vi "solar_type Set Value (ASCII).vi"(6 "ArrayDelimiters (1D,2D)":string[](array[string]), 7 "Keep Attributes? (F)":bool, 8 "error in (no error)":errorcluster, 10 "Value (ASCII)":string, 11 "Variant":variant) -> (0 "error out":errorcluster, 2 "Value (Binary)":string, 3 "Variant out":variant)   [LabVIEW 2018]
doc: "This sets the ASCII value into the Variant data."
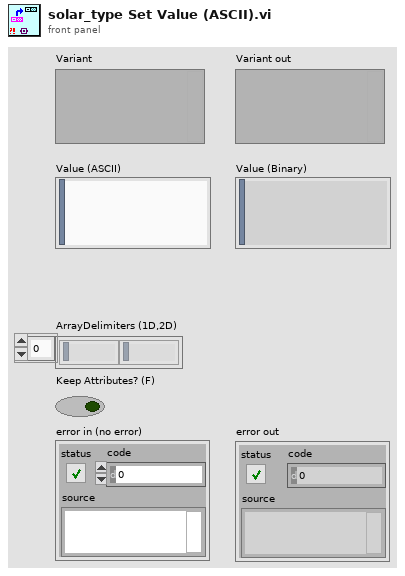
[diagram p1: front panel]
types:
  T1 = typedef "solar_type Item Type.ctl" = enum16{"NULL", "UNKNOWN", "CLUSTER", "I8", "I16", "I32", "I64", "U8", "U16", "U32", "U64", "U8_ENUM", "U16_ENUM", "U32_ENUM", "SGL", "DBL", "BOOLEAN", "STRING", "PATH", "VISA", "TAG", "TIME", "I8_1D", "I16_1D", "I32_1D", "I64_1D", "U8_1D", "U16_1D", "U32_1D", "U64_1D", "U8_ENUM_1D", "U16_ENUM_1D", "U32_ENUM_1D", "SGL_1D", "DBL_1D", "BOOLEAN_1D", "STRING_1D", "PATH_1D", "VISA_1D", "TAG_1D", "TIME_1D", "I8_2D", "I16_2D", "I32_2D", "I64_2D", "U8_2D", "U16_2D", "U32_2D", "U64_2D", "U8_ENUM_2D", "U16_ENUM_2D", "U32_ENUM_2D", "SGL_2D", "DBL_2D", "BOOLEAN_2D", "STRING_2D", "PATH_2D", "VISA_2D", "TAG_2D", "TIME_2D"}
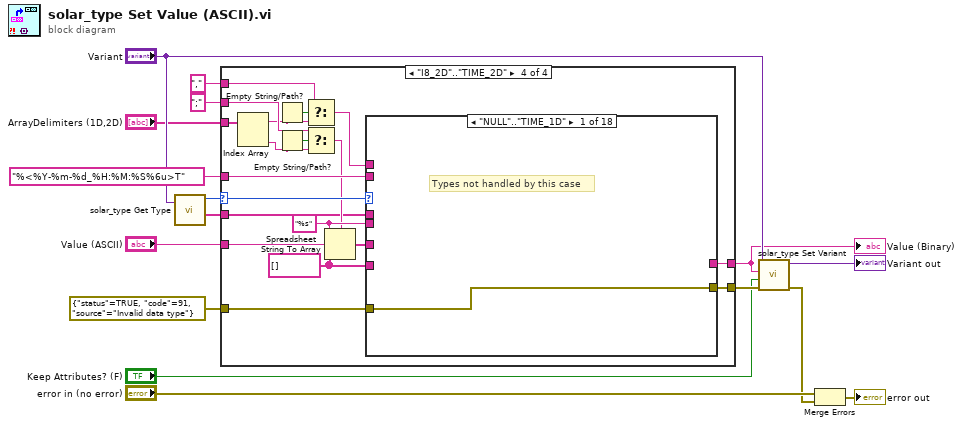
[diagram p0: block diagram]
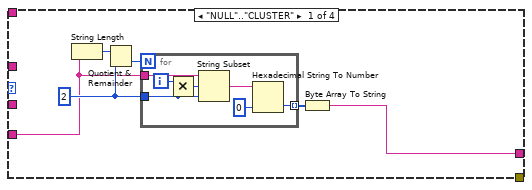
[diagram p2: hidden frame]
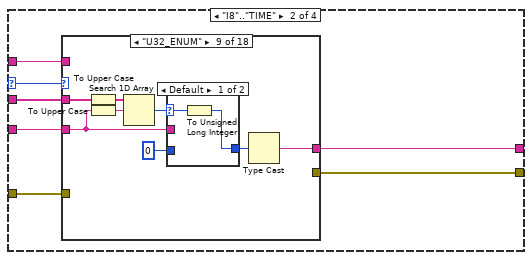
[diagram p3: hidden frame]
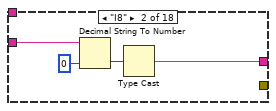
[diagram p5: hidden frame]
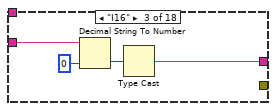
[diagram p6: hidden frame]
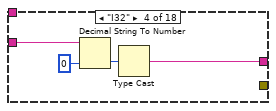
[diagram p7: hidden frame]
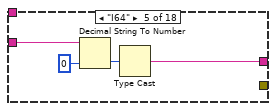
[diagram p8: hidden frame]
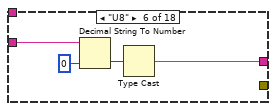
[diagram p9: hidden frame]
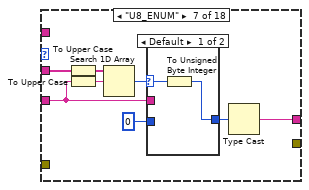
[diagram p10: hidden frame]
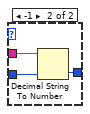
[diagram p11: hidden frame]
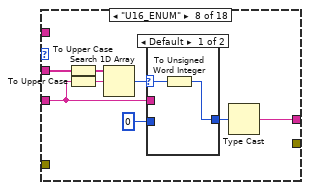
[diagram p12: hidden frame]
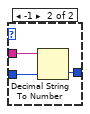
[diagram p13: hidden frame]
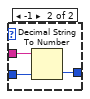
[diagram p14: hidden frame]
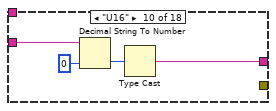
[diagram p15: hidden frame]
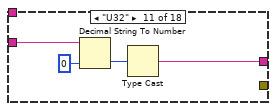
[diagram p16: hidden frame]
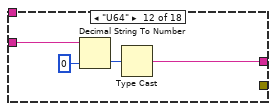
[diagram p17: hidden frame]
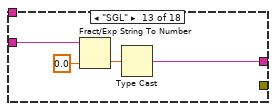
[diagram p18: hidden frame]
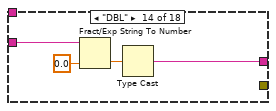
[diagram p19: hidden frame]
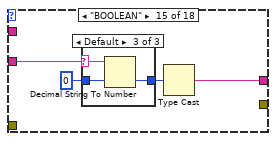
[diagram p20: hidden frame]
diagram:
  n1 = call "solar_type Get Type.vi"("Variant"="Variant") -> ("Type"=w11:T1, "Enum Names"=w3:string[])  [unwired: 4 in, 1 out]
  n2 = case shown="\"I8_2D\"..\"TIME_2D\"" w11 {
    selector: w11 -> [_ w36 w154 w300]
    tunnel: "Value (ASCII)" -> [w18 w31 w150 w299]
    tunnel: [_ w33 w151 w302] -> w10
    tunnel: [w17 w35 w153 w303] -> w1
    tunnel: errorcluster {"status"=TRUE, "code"=91, "source"="Invalid data type"} ("error in (no error)") -> [_ w34 w152 w301]
    tunnel: "%<%Y-%m-%d_%H:%M:%S%6u>T" -> [_ w32 w146 w298]
    tunnel: "," -> [_ _ w143 w295]
    tunnel: ";" -> [_ _ _ w292]
    tunnel: w3 -> [_ w30 w140 w288]
    tunnel: "ArrayDelimiters (1D,2D)" -> [_ _ w141 w290]
    frame "NULL".."CLUSTER" {
      w22 = 2 ("y")
      n3 = String Length(string=w18) -> (length=w20:i32)
      n4 = Quotient & Remainder(x=w20, y=w22) -> (floor(x/y)=w21:i32)  [unwired: 1 out]
      n5 = for {
        N: w21 -> [_]
        tunnel: w18 -> [w29]
        tunnel: [w24] -> w19 mode=indexing
        tunnel: w22 -> [w23]
        i -> [w28]
        n6 = Multiply(x=w28, y=w23) -> (x*y=w27:i32)
        n7 = String Subset(string=w29, offset (0)=w27, length (rest)=w23) -> (substring=w26:string)
        n8 = Hexadecimal String To Number(string=w26, default (0uL)=u8 0 ("default (0 U32)")) -> (number=w24:u8)  [unwired: 1 in, 1 out]
      }
      n9 = Byte Array To String(unsigned byte array=w19) -> (string=w17:string)
    }
    frame "I8".."TIME" {
      n10 = case shown="\"U32_ENUM\"" w36 {
        tunnel: w31 -> [_ w41 w45 w49 w53 w57 w62 w75 w88 w100 w104 w108 w112 w116 w120 w127 w131 w139]
        tunnel: [_ w38 w42 w46 w50 w54 w64 w77 w90 w97 w101 w105 w109 w113 w117 w126 w133 w134] -> w35
        tunnel: w34 -> [w37 _ _ _ _ _ _ _ _ _ _ _ _ _ _ _ _ _]
        tunnel: [w37 _ _ _ _ _ _ _ _ _ _ _ _ _ _ _ w132 w138] -> w33
        tunnel: w32 -> [_ _ _ _ _ _ _ _ _ _ _ _ _ _ _ _ _ w137]
        tunnel: w30 -> [_ _ _ _ _ _ w63 w76 w89 _ _ _ _ _ _ _ _ _]
        frame "NULL".."CLUSTER", "I8_1D".."TIME_2D" {
          # "Not handled by this case"
        }
        frame "I8" {
          n11 = Decimal String To Number(string=w41, default (0L)=i8 0 ("default (0 I32)")) -> (number=w39:i8)  [unwired: 1 in, 1 out]
          n12 = Type Cast(x=w39) -> (*(type *) &x=w38:string)  [unwired: 1 in]
        }
        frame "I16" {
          n13 = Decimal String To Number(string=w45, default (0L)=i16 0 ("default (0 I32)")) -> (number=w43:i16)  [unwired: 1 in, 1 out]
          n14 = Type Cast(x=w43) -> (*(type *) &x=w42:string)  [unwired: 1 in]
        }
        frame "I32" {
          n15 = Decimal String To Number(string=w49, default (0L)=0 ("default (0 I32)")) -> (number=w47:i32)  [unwired: 1 in, 1 out]
          n16 = Type Cast(x=w47) -> (*(type *) &x=w46:string)  [unwired: 1 in]
        }
        frame "I64" {
          n17 = Decimal String To Number(string=w53, default (0L)=i64 0 ("default (0 I32)")) -> (number=w51:i64)  [unwired: 1 in, 1 out]
          n18 = Type Cast(x=w51) -> (*(type *) &x=w50:string)  [unwired: 1 in]
        }
        frame "U8" {
          n19 = Decimal String To Number(string=w57, default (0L)=u8 0 ("default (0 I32)")) -> (number=w55:u8)  [unwired: 1 in, 1 out]
          n20 = Type Cast(x=w55) -> (*(type *) &x=w54:string)  [unwired: 1 in]
        }
        frame "U8_ENUM" {
          n21 = To Upper Case(1:w63) -> (0:w60:string[])
          n22 = To Upper Case(1:w62) -> (0:w59:string)
          n23 = Search 1D Array(1D array=w60, element=w59) -> (index of element=w61:i32)  [unwired: 1 in]
          n24 = case shown="Default" w61 {
            selector: w61 -> [w67 _]
            tunnel: [w66 w70] -> w65
            tunnel: w62 -> [_ w69]
            tunnel: u8 0 ("default (0 I32)") -> [_ w68]
            frame Default {
              n25 = To Unsigned Byte Integer(number=w67) -> (unsigned 8bit integer=w66:u8)
            }
            frame -1 {
              n26 = Decimal String To Number(string=w69, default (0L)=w68) -> (number=w70:u8)  [unwired: 1 in, 1 out]
            }
          }
          n27 = Type Cast(x=w65) -> (*(type *) &x=w64:string)  [unwired: 1 in]
        }
        frame "U16_ENUM" {
          n28 = To Upper Case(1:w76) -> (0:w73:string[])
          n29 = To Upper Case(1:w75) -> (0:w72:string)
          n30 = Search 1D Array(1D array=w73, element=w72) -> (index of element=w74:i32)  [unwired: 1 in]
          n31 = case shown="Default" w74 {
            selector: w74 -> [w80 _]
            tunnel: [w79 w83] -> w78
            tunnel: w75 -> [_ w82]
            tunnel: u16 0 ("default (0 I32)") -> [_ w81]
            frame Default {
              n32 = To Unsigned Word Integer(number=w80) -> (unsigned 16bit integer=w79:u16)
            }
            frame -1 {
              n33 = Decimal String To Number(string=w82, default (0L)=w81) -> (number=w83:u16)  [unwired: 1 in, 1 out]
            }
          }
          n34 = Type Cast(x=w78) -> (*(type *) &x=w77:string)  [unwired: 1 in]
        }
        frame "U32_ENUM" {
          n35 = To Upper Case(1:w89) -> (0:w86:string[])
          n36 = To Upper Case(1:w88) -> (0:w85:string)
          n37 = Search 1D Array(1D array=w86, element=w85) -> (index of element=w87:i32)  [unwired: 1 in]
          n38 = case shown="Default" w87 {
            selector: w87 -> [w93 _]
            tunnel: [w92 w96] -> w91
            tunnel: w88 -> [_ w95]
            tunnel: u32 0 ("default (0 I32)") -> [_ w94]
            frame Default {
              n39 = To Unsigned Long Integer(number=w93) -> (unsigned 32bit integer=w92:u32)
            }
            frame -1 {
              n40 = Decimal String To Number(string=w95, default (0L)=w94) -> (number=w96:u32)  [unwired: 1 in, 1 out]
            }
          }
          n41 = Type Cast(x=w91) -> (*(type *) &x=w90:string)  [unwired: 1 in]
        }
        frame "U16" {
          n42 = Decimal String To Number(string=w100, default (0L)=u16 0 ("default (0 I32)")) -> (number=w98:u16)  [unwired: 1 in, 1 out]
          n43 = Type Cast(x=w98) -> (*(type *) &x=w97:string)  [unwired: 1 in]
        }
        frame "U32" {
          n44 = Decimal String To Number(string=w104, default (0L)=u32 0 ("default (0 I32)")) -> (number=w102:u32)  [unwired: 1 in, 1 out]
          n45 = Type Cast(x=w102) -> (*(type *) &x=w101:string)  [unwired: 1 in]
        }
        frame "U64" {
          n46 = Decimal String To Number(string=w108, default (0L)=u64 0 ("default (0 I32)")) -> (number=w106:u64)  [unwired: 1 in, 1 out]
          n47 = Type Cast(x=w106) -> (*(type *) &x=w105:string)  [unwired: 1 in]
        }
        frame "SGL" {
          n48 = Fract/Exp String To Number(string=w112, default (0 dbl)=sgl 0.0 ("default (0 I32)")) -> (number=w110:sgl)  [unwired: 2 in, 1 out]
          n49 = Type Cast(x=w110) -> (*(type *) &x=w109:string)  [unwired: 1 in]
        }
        frame "DBL" {
          n50 = Fract/Exp String To Number(string=w116, default (0 dbl)=0.0 ("default (0 I32)")) -> (number=w114:dbl)  [unwired: 2 in, 1 out]
          n51 = Type Cast(x=w114) -> (*(type *) &x=w113:string)  [unwired: 1 in]
        }
        frame "BOOLEAN" {
          n52 = case shown="Default" w120 {
            selector: w120 -> [_ _ w125]
            tunnel: u8 0 ("default (0 I32)") -> [w121 _ w124]
            tunnel: [w121 u8 1 w123] -> w118
            frame "false" {
            }
            frame "true" {
            }
            frame Default {
              n53 = Decimal String To Number(string=w125, default (0L)=w124) -> (number=w123:u8)  [unwired: 1 in, 1 out]
            }
          }
          n54 = Type Cast(x=w118) -> (*(type *) &x=w117:string)  [unwired: 1 in]
        }
        frame "STRING", "VISA", "TAG" {
          n55 = String Length(string=w127) -> (length=w129:i32)
          n56 = Type Cast(x=w129) -> (*(type *) &x=w128:string)  [unwired: 1 in]
          n57 = Concatenate Strings(w128, w127) -> (w126:string)
        }
        frame "PATH" {
          # "PTH0<I32_size>..."
          n58 = String To Path(string=w131) -> (path=w130:path)
          n59 = Flatten To String(anything=w130) -> (data string=w133:string, error out=w132:errorcluster)  [unwired: 3 in, 1 out]
        }
        frame "TIME" {
          # "16 bytes"
          n60 = Scan From String(format string=w137, input string=w139, default 1=timestamp(0 s since 1904-01-01)) -> (error out=w138:errorcluster, output 1=w135:timestamp)  [unwired: 2 in, 2 out]
          n61 = Flatten To String(anything=w135) -> (data string=w134:string)  [unwired: 3 in, 2 out]
        }
      }
    }
    frame "I8_1D".."TIME_1D" {
      n62 = Index Array(array=w141) -> (element=w142:string)  [unwired: 1 in]
      n63 = Empty String/Path?(string/path=w142) -> (empty?=w145:bool)
      n64 = Select(t=w143, s=w145, f=w142) -> (s? t:f=w144:string)
      n65 = Spreadsheet String To Array(delimiter (Tab)=w144, format string="%s", spreadsheet string=w150, array type (2D Dbl)=string[] []) -> (array=w147:string[])
      n66 = case shown="\"U32_ENUM_1D\"" w154 {
        tunnel: w147 -> [_ w158 w163 w168 w173 w178 w183 w188 w193 w197 w214 w231 w249 w254 w260 w269 w273 w280]
        tunnel: [_ w160 w165 w170 w175 w180 w185 w190 w195 w201 w218 w235 w251 w256 w258 w271 w275 w281] -> w153
        tunnel: w152 -> [w155 _ _ _ _ _ _ _ _ _ _ _ _ _ _ _ _ _]
        tunnel: [w155 w159 w164 w169 w174 w179 w184 w189 w194 w200 w217 w234 w250 w255 w257 w270 w274 w279] -> w151
        tunnel: w146 -> [_ _ _ _ _ _ _ _ _ _ _ _ _ _ _ _ _ w278]
        tunnel: w140 -> [_ _ _ _ _ _ _ _ _ w198 w215 w232 _ _ _ _ _ _]
        frame "NULL".."TIME", "I8_2D".."TIME_2D" {
        }
        frame "I8_1D" {
          n67 = Decimal String To Number(string=w158, default (0L)=i8 0 ("default (0 I32)")) -> (number=w156:i8[])  [unwired: 1 in, 1 out]
          n68 = Flatten To String(anything=w156) -> (data string=w160:string, error out=w159:errorcluster)  [unwired: 3 in, 1 out]
        }
        frame "I16_1D" {
          n69 = Decimal String To Number(string=w163, default (0L)=i16 0 ("default (0 I32)")) -> (number=w161:i16[])  [unwired: 1 in, 1 out]
          n70 = Flatten To String(anything=w161) -> (data string=w165:string, error out=w164:errorcluster)  [unwired: 3 in, 1 out]
        }
        frame "I32_1D" {
          n71 = Decimal String To Number(string=w168, default (0L)=0 ("default (0 I32)")) -> (number=w166:i32[])  [unwired: 1 in, 1 out]
          n72 = Flatten To String(anything=w166) -> (data string=w170:string, error out=w169:errorcluster)  [unwired: 3 in, 1 out]
        }
        frame "I64_1D" {
          n73 = Decimal String To Number(string=w173, default (0L)=i64 0 ("default (0 I32)")) -> (number=w171:i64[])  [unwired: 1 in, 1 out]
          n74 = Flatten To String(anything=w171) -> (data string=w175:string, error out=w174:errorcluster)  [unwired: 3 in, 1 out]
        }
        frame "U8_1D" {
          n75 = Decimal String To Number(string=w178, default (0L)=u8 0 ("default (0 I32)")) -> (number=w176:u8[])  [unwired: 1 in, 1 out]
          n76 = Flatten To String(anything=w176) -> (data string=w180:string, error out=w179:errorcluster)  [unwired: 3 in, 1 out]
        }
        frame "U16_1D" {
          n77 = Decimal String To Number(string=w183, default (0L)=u16 0 ("default (0 I32)")) -> (number=w181:u16[])  [unwired: 1 in, 1 out]
          n78 = Flatten To String(anything=w181) -> (data string=w185:string, error out=w184:errorcluster)  [unwired: 3 in, 1 out]
        }
        frame "U32_1D" {
          n79 = Decimal String To Number(string=w188, default (0L)=u32 0 ("default (0 I32)")) -> (number=w186:u32[])  [unwired: 1 in, 1 out]
          n80 = Flatten To String(anything=w186) -> (data string=w190:string, error out=w189:errorcluster)  [unwired: 3 in, 1 out]
        }
        frame "U64_1D" {
          n81 = Decimal String To Number(string=w193, default (0L)=u64 0 ("default (0 I32)")) -> (number=w191:u64[])  [unwired: 1 in, 1 out]
          n82 = Flatten To String(anything=w191) -> (data string=w195:string, error out=w194:errorcluster)  [unwired: 3 in, 1 out]
        }
        frame "U8_ENUM_1D" {
          n83 = To Upper Case(1:w198) -> (0:w199:string[])
          n84 = for {
            tunnel: w199 -> [w206]
            tunnel: w197 -> [w203] mode=indexing
            tunnel: [w204] -> w196 mode=indexing
            n85 = To Upper Case(1:w203) -> (0:w202:string)
            n86 = Search 1D Array(1D array=w206, element=w202) -> (index of element=w207:i32)  [unwired: 1 in]
            n87 = case shown="Default" w207 {
              selector: w207 -> [w209 _]
              tunnel: [w208 w212] -> w204
              tunnel: w203 -> [_ w211]
              tunnel: u8 0 ("default (0 I32)") -> [_ w210]
              frame Default {
                n88 = To Unsigned Byte Integer(number=w209) -> (unsigned 8bit integer=w208:u8)
              }
              frame -1 {
                n89 = Decimal String To Number(string=w211, default (0L)=w210) -> (number=w212:u8)  [unwired: 1 in, 1 out]
              }
            }
          }
          n90 = Flatten To String(anything=w196) -> (data string=w201:string, error out=w200:errorcluster)  [unwired: 3 in, 1 out]
        }
        frame "U16_ENUM_1D" {
          n91 = To Upper Case(1:w215) -> (0:w216:string[])
          n92 = for {
            tunnel: w216 -> [w223]
            tunnel: w214 -> [w220] mode=indexing
            tunnel: [w221] -> w213 mode=indexing
            n93 = To Upper Case(1:w220) -> (0:w219:string)
            n94 = Search 1D Array(1D array=w223, element=w219) -> (index of element=w224:i32)  [unwired: 1 in]
            n95 = case shown="Default" w224 {
              selector: w224 -> [w226 _]
              tunnel: [w225 w229] -> w221
              tunnel: w220 -> [_ w228]
              tunnel: u16 0 ("default (0 I32)") -> [_ w227]
              frame Default {
                n96 = To Unsigned Word Integer(number=w226) -> (unsigned 16bit integer=w225:u16)
              }
              frame -1 {
                n97 = Decimal String To Number(string=w228, default (0L)=w227) -> (number=w229:u16)  [unwired: 1 in, 1 out]
              }
            }
          }
          n98 = Flatten To String(anything=w213) -> (data string=w218:string, error out=w217:errorcluster)  [unwired: 3 in, 1 out]
        }
        frame "U32_ENUM_1D" {
          n99 = To Upper Case(1:w232) -> (0:w233:string[])
          n100 = for {
            tunnel: w233 -> [w240]
            tunnel: w231 -> [w237] mode=indexing
            tunnel: [w238] -> w230 mode=indexing
            n101 = To Upper Case(1:w237) -> (0:w236:string)
            n102 = Search 1D Array(1D array=w240, element=w236) -> (index of element=w241:i32)  [unwired: 1 in]
            n103 = case shown="Default" w241 {
              selector: w241 -> [w243 _]
              tunnel: [w242 w246] -> w238
              tunnel: w237 -> [_ w245]
              tunnel: u32 0 ("default (0 I32)") -> [_ w244]
              frame Default {
                n104 = To Unsigned Long Integer(number=w243) -> (unsigned 32bit integer=w242:u32)
              }
              frame -1 {
                n105 = Decimal String To Number(string=w245, default (0L)=w244) -> (number=w246:u32)  [unwired: 1 in, 1 out]
              }
            }
          }
          n106 = Flatten To String(anything=w230) -> (data string=w235:string, error out=w234:errorcluster)  [unwired: 3 in, 1 out]
        }
        frame "SGL_1D" {
          n107 = Fract/Exp String To Number(string=w249, default (0 dbl)=sgl 0.0 ("default (0 I32)")) -> (number=w247:sgl[])  [unwired: 2 in, 1 out]
          n108 = Flatten To String(anything=w247) -> (data string=w251:string, error out=w250:errorcluster)  [unwired: 3 in, 1 out]
        }
        frame "DBL_1D" {
          n109 = Fract/Exp String To Number(string=w254, default (0 dbl)=0.0 ("default (0 I32)")) -> (number=w252:dbl[])  [unwired: 2 in, 1 out]
          n110 = Flatten To String(anything=w252) -> (data string=w256:string, error out=w255:errorcluster)  [unwired: 3 in, 1 out]
        }
        frame "BOOLEAN_1D" {
          n111 = for {
            tunnel: w260 -> [w263] mode=indexing
            tunnel: [w262] -> w259 mode=indexing
            n112 = case shown="Default" w263 {
              selector: w263 -> [_ _ w268]
              tunnel: u8 0 ("default (0 I32)") -> [w264 _ w267]
              tunnel: [w264 u8 1 w266] -> w262
              frame "false" {
              }
              frame "true" {
              }
              frame Default {
                n113 = Decimal String To Number(string=w268, default (0L)=w267) -> (number=w266:u8)  [unwired: 1 in, 1 out]
              }
            }
          }
          n114 = Flatten To String(anything=w259) -> (data string=w258:string, error out=w257:errorcluster)  [unwired: 3 in, 1 out]
        }
        frame "STRING_1D", "VISA_1D", "TAG_1D" {
          n115 = Flatten To String(anything=w269) -> (data string=w271:string, error out=w270:errorcluster)  [unwired: 3 in, 1 out]
        }
        frame "PATH_1D" {
          n116 = String To Path(string=w273) -> (path=w272:path[])
          n117 = Flatten To String(anything=w272) -> (data string=w275:string, error out=w274:errorcluster)  [unwired: 3 in, 1 out]
        }
        frame "TIME_1D" {
          n118 = for {
            tunnel: w280 -> [w287] mode=indexing
            tunnel: w278 -> [w284]
            shift-right: [w285] -> w279
            shift-left: _ -> [w286]
            tunnel: timestamp(0 s since 1904-01-01) -> [w283]
            tunnel: [w282] -> w276 mode=indexing
            n119 = Scan From String(format string=w284, input string=w287, error in=w286, default 1=w283) -> (error out=w285:errorcluster, output 1=w282:timestamp)  [unwired: 1 in, 2 out]
          }
          n120 = Flatten To String(anything=w276) -> (data string=w281:string)  [unwired: 3 in, 2 out]
        }
      }
    }
    frame "I8_2D".."TIME_2D" {
      w305 = string[] []
      w304 = "%s" ("format string")
      n121 = Index Array(array=w290) -> (element #1=w291:string, element #2=w289:string)  [unwired: 2 in]
      n122 = Empty String/Path?(string/path=w291) -> (empty?=w297:bool)
      n123 = Empty String/Path?(string/path=w289) -> (empty?=w294:bool)
      n124 = Select(t=w295, s=w297, f=w291) -> (s? t:f=w296:string)
      n125 = Select(t=w292, s=w294, f=w289) -> (s? t:f=w293:string)
      n126 = Spreadsheet String To Array(delimiter (Tab)=w293, format string=w304, spreadsheet string=w299, array type (2D Dbl)=w305) -> (array=w306:string[])
      n127 = case shown="\"NULL\"..\"TIME_1D\"" w300 {
        tunnel: w306 -> [_ w314 w328 w342 w356 w370 w384 w398 w412 w427 w454 w481 w507 w521 w535 w556 w568 w582]
        tunnel: w305 -> [_ w313 w327 w341 w355 w369 w383 w397 w411 w426 w453 w480 w506 w520 w534 w555 w567 w581]
        tunnel: w304 -> [_ w312 w326 w340 w354 w368 w382 w396 w410 w425 w452 w479 w505 w519 w533 w554 w566 w580]
        tunnel: w296 -> [_ w311 w325 w339 w353 w367 w381 w395 w409 w424 w451 w478 w504 w518 w532 w553 w565 w579]
        tunnel: [_ w310 w323 w337 w351 w365 w379 w393 w407 w422 w449 w476 w502 w516 w530 w551 w563 w578] -> w303
        tunnel: [w307 w309 w322 w336 w350 w364 w378 w392 w406 w421 w448 w475 w501 w515 w529 w550 w562 w576] -> w302
        tunnel: w301 -> [w307 _ _ _ _ _ _ _ _ _ _ _ _ _ _ _ _ _]
        tunnel: w298 -> [_ _ _ _ _ _ _ _ _ _ _ _ _ _ _ _ _ w575]
        tunnel: w288 -> [_ _ _ _ _ _ _ _ _ w420 w447 w474 _ _ _ _ _ _]
        frame "NULL".."TIME_1D" {
          # "Types not handled by this case"
        }
        frame "I8_2D" {
          n128 = for {
            tunnel: w314 -> [w321] mode=indexing
            tunnel: w313 -> [w320]
            tunnel: w312 -> [w319]
            tunnel: w311 -> [w318]
            tunnel: [w316] -> w308 mode=indexing
            n129 = Spreadsheet String To Array(delimiter (Tab)=w318, format string=w319, spreadsheet string=w321, array type (2D Dbl)=w320) -> (array=w317:string[])
            n130 = Decimal String To Number(string=w317, default (0L)=i8 0) -> (number=w316:i8[])  [unwired: 1 in, 1 out]
          }
          n131 = Flatten To String(anything=w308) -> (data string=w310:string, error out=w309:errorcluster)  [unwired: 3 in, 1 out]
        }
        frame "I16_2D" {
          n132 = for {
            tunnel: w328 -> [w335] mode=indexing
            tunnel: w327 -> [w334]
            tunnel: w326 -> [w333]
            tunnel: w325 -> [w332]
            tunnel: [w330] -> w324 mode=indexing
            n133 = Spreadsheet String To Array(delimiter (Tab)=w332, format string=w333, spreadsheet string=w335, array type (2D Dbl)=w334) -> (array=w331:string[])
            n134 = Decimal String To Number(string=w331, default (0L)=i16 0) -> (number=w330:i16[])  [unwired: 1 in, 1 out]
          }
          n135 = Flatten To String(anything=w324) -> (data string=w323:string, error out=w322:errorcluster)  [unwired: 3 in, 1 out]
        }
        frame "I32_2D" {
          n136 = for {
            tunnel: w342 -> [w349] mode=indexing
            tunnel: w341 -> [w348]
            tunnel: w340 -> [w347]
            tunnel: w339 -> [w346]
            tunnel: [w344] -> w338 mode=indexing
            n137 = Spreadsheet String To Array(delimiter (Tab)=w346, format string=w347, spreadsheet string=w349, array type (2D Dbl)=w348) -> (array=w345:string[])
            n138 = Decimal String To Number(string=w345, default (0L)=0) -> (number=w344:i32[])  [unwired: 1 in, 1 out]
          }
          n139 = Flatten To String(anything=w338) -> (data string=w337:string, error out=w336:errorcluster)  [unwired: 3 in, 1 out]
        }
        frame "I64_2D" {
          n140 = for {
            tunnel: w356 -> [w363] mode=indexing
            tunnel: w355 -> [w362]
            tunnel: w354 -> [w361]
            tunnel: w353 -> [w360]
            tunnel: [w358] -> w352 mode=indexing
            n141 = Spreadsheet String To Array(delimiter (Tab)=w360, format string=w361, spreadsheet string=w363, array type (2D Dbl)=w362) -> (array=w359:string[])
            n142 = Decimal String To Number(string=w359, default (0L)=i64 0) -> (number=w358:i64[])  [unwired: 1 in, 1 out]
          }
          n143 = Flatten To String(anything=w352) -> (data string=w351:string, error out=w350:errorcluster)  [unwired: 3 in, 1 out]
        }
        frame "U8_2D" {
          n144 = for {
            tunnel: w370 -> [w377] mode=indexing
            tunnel: w369 -> [w376]
            tunnel: w368 -> [w375]
            tunnel: w367 -> [w374]
            tunnel: [w372] -> w366 mode=indexing
            n145 = Spreadsheet String To Array(delimiter (Tab)=w374, format string=w375, spreadsheet string=w377, array type (2D Dbl)=w376) -> (array=w373:string[])
            n146 = Decimal String To Number(string=w373, default (0L)=u8 0) -> (number=w372:u8[])  [unwired: 1 in, 1 out]
          }
          n147 = Flatten To String(anything=w366) -> (data string=w365:string, error out=w364:errorcluster)  [unwired: 3 in, 1 out]
        }
        frame "U16_2D" {
          n148 = for {
            tunnel: w384 -> [w391] mode=indexing
            tunnel: w383 -> [w390]
            tunnel: w382 -> [w389]
            tunnel: w381 -> [w388]
            tunnel: [w386] -> w380 mode=indexing
            n149 = Spreadsheet String To Array(delimiter (Tab)=w388, format string=w389, spreadsheet string=w391, array type (2D Dbl)=w390) -> (array=w387:string[])
            n150 = Decimal String To Number(string=w387, default (0L)=u16 0) -> (number=w386:u16[])  [unwired: 1 in, 1 out]
          }
          n151 = Flatten To String(anything=w380) -> (data string=w379:string, error out=w378:errorcluster)  [unwired: 3 in, 1 out]
        }
        frame "U32_2D" {
          n152 = for {
            tunnel: w398 -> [w405] mode=indexing
            tunnel: w397 -> [w404]
            tunnel: w396 -> [w403]
            tunnel: w395 -> [w402]
            tunnel: [w400] -> w394 mode=indexing
            n153 = Spreadsheet String To Array(delimiter (Tab)=w402, format string=w403, spreadsheet string=w405, array type (2D Dbl)=w404) -> (array=w401:string[])
            n154 = Decimal String To Number(string=w401, default (0L)=u32 0) -> (number=w400:u32[])  [unwired: 1 in, 1 out]
          }
          n155 = Flatten To String(anything=w394) -> (data string=w393:string, error out=w392:errorcluster)  [unwired: 3 in, 1 out]
        }
        frame "U64_2D" {
          n156 = for {
            tunnel: w412 -> [w419] mode=indexing
            tunnel: w411 -> [w418]
            tunnel: w410 -> [w417]
            tunnel: w409 -> [w416]
            tunnel: [w414] -> w408 mode=indexing
            n157 = Spreadsheet String To Array(delimiter (Tab)=w416, format string=w417, spreadsheet string=w419, array type (2D Dbl)=w418) -> (array=w415:string[])
            n158 = Decimal String To Number(string=w415, default (0L)=u64 0) -> (number=w414:u64[])  [unwired: 1 in, 1 out]
          }
          n159 = Flatten To String(anything=w408) -> (data string=w407:string, error out=w406:errorcluster)  [unwired: 3 in, 1 out]
        }
        frame "U8_ENUM_2D" {
          n160 = for {
            tunnel: w427 -> [w435] mode=indexing
            tunnel: w426 -> [w434]
            tunnel: w425 -> [w433]
            tunnel: w424 -> [w432]
            tunnel: [w428] -> w423 mode=indexing
            tunnel: w420 -> [w429]
            n161 = Spreadsheet String To Array(delimiter (Tab)=w432, format string=w433, spreadsheet string=w435, array type (2D Dbl)=w434) -> (array=w430:string[])
            n162 = To Upper Case(1:w429) -> (0:w431:string[])
            n163 = for {
              tunnel: w431 -> [w440]
              tunnel: w430 -> [w437] mode=indexing
              tunnel: [w438] -> w428 mode=indexing
              n164 = To Upper Case(1:w437) -> (0:w436:string)
              n165 = Search 1D Array(1D array=w440, element=w436) -> (index of element=w441:i32)  [unwired: 1 in]
              n166 = case shown="Default" w441 {
                selector: w441 -> [w443 _]
                tunnel: [w442 w446] -> w438
                tunnel: w437 -> [_ w445]
                tunnel: u8 0 ("default (0 I32)") -> [_ w444]
                frame Default {
                  n167 = To Unsigned Byte Integer(number=w443) -> (unsigned 8bit integer=w442:u8)
                }
                frame -1 {
                  n168 = Decimal String To Number(string=w445, default (0L)=w444) -> (number=w446:u8)  [unwired: 1 in, 1 out]
                }
              }
            }
          }
          n169 = Flatten To String(anything=w423) -> (data string=w422:string, error out=w421:errorcluster)  [unwired: 3 in, 1 out]
        }
        frame "U16_ENUM_2D" {
          n170 = for {
            tunnel: w454 -> [w462] mode=indexing
            tunnel: w453 -> [w461]
            tunnel: w452 -> [w460]
            tunnel: w451 -> [w459]
            tunnel: [w455] -> w450 mode=indexing
            tunnel: w447 -> [w456]
            n171 = Spreadsheet String To Array(delimiter (Tab)=w459, format string=w460, spreadsheet string=w462, array type (2D Dbl)=w461) -> (array=w457:string[])
            n172 = To Upper Case(1:w456) -> (0:w458:string[])
            n173 = for {
              tunnel: w458 -> [w467]
              tunnel: w457 -> [w464] mode=indexing
              tunnel: [w465] -> w455 mode=indexing
              n174 = To Upper Case(1:w464) -> (0:w463:string)
              n175 = Search 1D Array(1D array=w467, element=w463) -> (index of element=w468:i32)  [unwired: 1 in]
              n176 = case shown="Default" w468 {
                selector: w468 -> [w470 _]
                tunnel: [w469 w473] -> w465
                tunnel: w464 -> [_ w472]
                tunnel: u16 0 ("default (0 I32)") -> [_ w471]
                frame Default {
                  n177 = To Unsigned Word Integer(number=w470) -> (unsigned 16bit integer=w469:u16)
                }
                frame -1 {
                  n178 = Decimal String To Number(string=w472, default (0L)=w471) -> (number=w473:u16)  [unwired: 1 in, 1 out]
                }
              }
            }
          }
          n179 = Flatten To String(anything=w450) -> (data string=w449:string, error out=w448:errorcluster)  [unwired: 3 in, 1 out]
        }
        frame "U32_ENUM_2D" {
          n180 = for {
            tunnel: w481 -> [w489] mode=indexing
            tunnel: w480 -> [w488]
            tunnel: w479 -> [w487]
            tunnel: w478 -> [w486]
            tunnel: [w482] -> w477 mode=indexing
            tunnel: w474 -> [w483]
            n181 = Spreadsheet String To Array(delimiter (Tab)=w486, format string=w487, spreadsheet string=w489, array type (2D Dbl)=w488) -> (array=w484:string[])
            n182 = To Upper Case(1:w483) -> (0:w485:string[])
            n183 = for {
              tunnel: w485 -> [w494]
              tunnel: w484 -> [w491] mode=indexing
              tunnel: [w492] -> w482 mode=indexing
              n184 = To Upper Case(1:w491) -> (0:w490:string)
              n185 = Search 1D Array(1D array=w494, element=w490) -> (index of element=w495:i32)  [unwired: 1 in]
              n186 = case shown="Default" w495 {
                selector: w495 -> [w497 _]
                tunnel: [w496 w500] -> w492
                tunnel: w491 -> [_ w499]
                tunnel: u32 0 ("default (0 I32)") -> [_ w498]
                frame Default {
                  n187 = To Unsigned Long Integer(number=w497) -> (unsigned 32bit integer=w496:u32)
                }
                frame -1 {
                  n188 = Decimal String To Number(string=w499, default (0L)=w498) -> (number=w500:u32)  [unwired: 1 in, 1 out]
                }
              }
            }
          }
          n189 = Flatten To String(anything=w477) -> (data string=w476:string, error out=w475:errorcluster)  [unwired: 3 in, 1 out]
        }
        frame "SGL_2D" {
          n190 = for {
            tunnel: w507 -> [w514] mode=indexing
            tunnel: w506 -> [w513]
            tunnel: w505 -> [w512]
            tunnel: w504 -> [w511]
            tunnel: [w508] -> w503 mode=indexing
            n191 = Spreadsheet String To Array(delimiter (Tab)=w511, format string=w512, spreadsheet string=w514, array type (2D Dbl)=w513) -> (array=w510:string[])
            n192 = Fract/Exp String To Number(string=w510, default (0 dbl)=sgl 0.0) -> (number=w508:sgl[])  [unwired: 2 in, 1 out]
          }
          n193 = Flatten To String(anything=w503) -> (data string=w502:string, error out=w501:errorcluster)  [unwired: 3 in, 1 out]
        }
        frame "DBL_2D" {
          n194 = for {
            tunnel: w521 -> [w528] mode=indexing
            tunnel: w520 -> [w527]
            tunnel: w519 -> [w526]
            tunnel: w518 -> [w525]
            tunnel: [w522] -> w517 mode=indexing
            n195 = Spreadsheet String To Array(delimiter (Tab)=w525, format string=w526, spreadsheet string=w528, array type (2D Dbl)=w527) -> (array=w524:string[])
            n196 = Fract/Exp String To Number(string=w524, default (0 dbl)=0.0) -> (number=w522:dbl[])  [unwired: 2 in, 1 out]
          }
          n197 = Flatten To String(anything=w517) -> (data string=w516:string, error out=w515:errorcluster)  [unwired: 3 in, 1 out]
        }
        frame "BOOLEAN_2D" {
          n198 = for {
            tunnel: w535 -> [w541] mode=indexing
            tunnel: w534 -> [w540]
            tunnel: w533 -> [w539]
            tunnel: w532 -> [w538]
            tunnel: [w537] -> w531 mode=indexing
            n199 = Spreadsheet String To Array(delimiter (Tab)=w538, format string=w539, spreadsheet string=w541, array type (2D Dbl)=w540) -> (array=w536:string[])
            n200 = for {
              tunnel: w536 -> [w544] mode=indexing
              tunnel: [w543] -> w537 mode=indexing
              n201 = case shown="Default" w544 {
                selector: w544 -> [_ _ w549]
                tunnel: u8 0 ("default (0 I32)") -> [w545 _ w548]
                tunnel: [w545 u8 1 w547] -> w543
                frame "false" {
                }
                frame "true" {
                }
                frame Default {
                  n202 = Decimal String To Number(string=w549, default (0L)=w548) -> (number=w547:u8)  [unwired: 1 in, 1 out]
                }
              }
            }
          }
          n203 = Flatten To String(anything=w531) -> (data string=w530:string, error out=w529:errorcluster)  [unwired: 3 in, 1 out]
        }
        frame "STRING_2D", "VISA_2D", "TAG_2D" {
          n204 = for {
            tunnel: w556 -> [w561] mode=indexing
            tunnel: w555 -> [w560]
            tunnel: w554 -> [w559]
            tunnel: w553 -> [w558]
            tunnel: [w557] -> w552 mode=indexing
            n205 = Spreadsheet String To Array(delimiter (Tab)=w558, format string=w559, spreadsheet string=w561, array type (2D Dbl)=w560) -> (array=w557:string[])
          }
          n206 = Flatten To String(anything=w552) -> (data string=w551:string, error out=w550:errorcluster)  [unwired: 3 in, 1 out]
        }
        frame "PATH_2D" {
          n207 = for {
            tunnel: w568 -> [w574] mode=indexing
            tunnel: w567 -> [w573]
            tunnel: w566 -> [w572]
            tunnel: w565 -> [w571]
            tunnel: [w569] -> w564 mode=indexing
            n208 = Spreadsheet String To Array(delimiter (Tab)=w571, format string=w572, spreadsheet string=w574, array type (2D Dbl)=w573) -> (array=w570:string[])
            n209 = String To Path(string=w570) -> (path=w569:path[])
          }
          n210 = Flatten To String(anything=w564) -> (data string=w563:string, error out=w562:errorcluster)  [unwired: 3 in, 1 out]
        }
        frame "TIME_2D" {
          n211 = for {
            tunnel: w582 -> [w592] mode=indexing
            tunnel: w581 -> [w591]
            tunnel: w580 -> [w590]
            tunnel: w579 -> [w589]
            shift-right: [w586] -> w576
            shift-left: _ -> [w587]
            tunnel: [w585] -> w577 mode=indexing
            tunnel: w575 -> [w584]
            n212 = Spreadsheet String To Array(delimiter (Tab)=w589, format string=w590, spreadsheet string=w592, array type (2D Dbl)=w591) -> (array=w588:string[])
            n213 = for {
              tunnel: w588 -> [w598] mode=indexing
              tunnel: w584 -> [w595]
              shift-right: [w596] -> w586
              shift-left: w587 -> [w597]
              tunnel: timestamp(0 s since 1904-01-01) -> [w594]
              tunnel: [w593] -> w585 mode=indexing
              n214 = Scan From String(format string=w595, input string=w598, error in=w597, default 1=w594) -> (error out=w596:errorcluster, output 1=w593:timestamp)  [unwired: 1 in, 2 out]
            }
          }
          n215 = Flatten To String(anything=w577) -> (data string=w578:string)  [unwired: 3 in, 2 out]
        }
      }
    }
  }
  "Value (Binary)" <- w1
  n216 = call "solar_type Set Variant.vi"("error in (no error)"=w10, "Keep Attributes? (F)"="Keep Attributes? (F)", "Data String"=w1, "Variant in"="Variant") -> ("error out"=w6:errorcluster, "Variant out"=→"Variant out":variant)  [unwired: 5 in, 1 out]
  n217 = Merge Errors("error in (no error)", w6) -> (→"error out":errorcluster)
